vi "Accel Plugin Ref.vi"() -> (1 "Command Index":cluster{i32, i32}, 2 "Plugin VI Ref":refnum<vi>, 3 "Device Type":string)   [LabVIEW 2019]
uses:
  Accel Update Ops.ctl
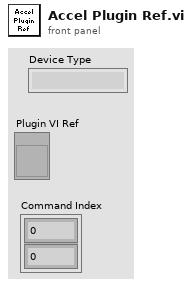
[diagram p1: front panel]
types:
  T1 = typedef "Accel Update Ops.ctl" = enum16{"get", "delete", "JSON update", "set  name", "transmit initial", "reset", "set init", "set range"}
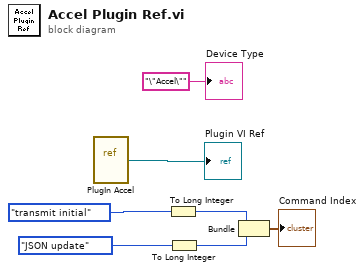
[diagram p0: block diagram]
diagram:
  n1 = vi-ref "PlugIn Accel.vi"() -> (→"Plugin VI Ref":refnum<vi>)
  n2 = To Long Integer(number=Accel_Update_Ops."transmit initial" ("menu")) -> (32bit integer=w3:i32)
  n3 = To Long Integer(number=Accel_Update_Ops."JSON update" ("menu")) -> (32bit integer=w2:i32)
  n4 = Bundle(w3, w2) -> (→"Command Index":cluster{i32, i32})  [unwired: 1 in]
  "Device Type" <- "\"Accel\""
